vi "1 bit errorr (SubVI).vi"(1 "Numeric":dbl, 2 "R in":bool[](array[boolean])) -> (0 "R out":bool[](array[boolean]))   [LabVIEW 2014]
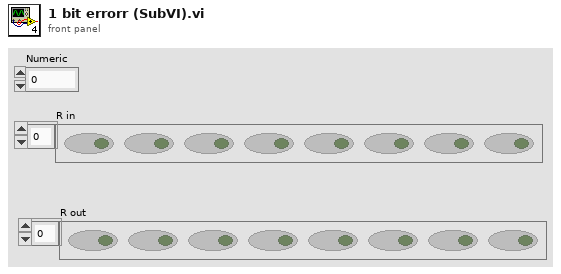
[diagram p1: front panel]
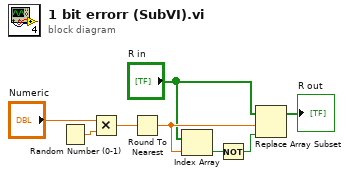
[diagram p0: block diagram]
diagram:
  n1 = Random Number (0-1)() -> (number: 0 to 1=w4:dbl)
  n2 = Multiply(x="Numeric", y=w4) -> (x*y=w5:dbl)
  n3 = Round To Nearest(number=w5) -> (nearest integer value=w6:dbl)
  n4 = Index Array(array="R in", index=w6) -> (element=w7:bool)
  n5 = Not(x=w7) -> (.not. x?=w8:bool)
  n6 = Replace Array Subset(array="R in", new element=w8, index=w6) -> (→"R out":bool[])
